vi "Receive notifier.vi"(10 "Variant":variant, 11 "notifier in":refnum<notifier>) -> (1 "message":string, 2 "data":variant, 3 "notifier out":refnum<notifier>)   [LabVIEW 2020]
uses:
  _controls/Notifier Cluster.ctl
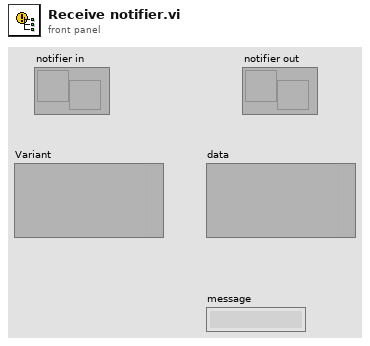
[diagram p1: front panel]
types:
  T1 = typedef "Notifier Cluster.ctl" = cluster{"message":string, "data":variant}
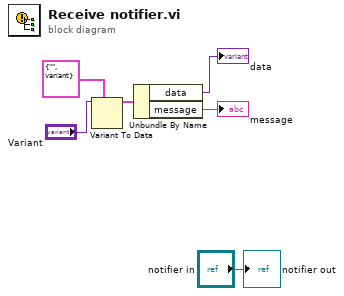
[diagram p0: block diagram]
diagram:
  n1 = Variant To Data(type=T1 {"message"="", "data"=variant}, Variant="Variant") -> (data=w3:T1)  [unwired: 1 in, 1 out]
  n2 = Unbundle By Name(w3) -> ("data"=→"data":variant, "message"=→"message":string)
  "notifier out" <- "notifier in"
